vi "Export.vi"(8 "error in (no error)":errorcluster, 11 "Test Report in":refnum<class "Test Report.Event.lvclass">) -> (0 "error out":errorcluster, 3 "Test Report out":refnum<class "Test Report.Event.lvclass">)   [LabVIEW 2020, in "Caraya.lvlib" / "Test Report.Event.lvclass"]
uses:
  Test Report.Event.lvclass
  C:/projects/caraya/src/classes/Test Report/Test Report.lvclass
  Test Report.Event.lvclass/Test Report.Event.ctl
  Test Report/Test Report.lvclass
  Test Result/Test Result.lvclass
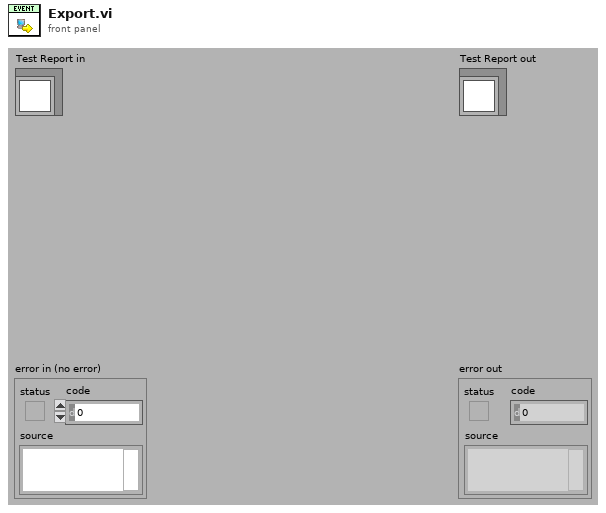
[diagram p1: front panel]
types:
  T1 = typedef "Caraya.lvlib/Test Result.lvclass/Node Results (Extended).ctl" = cluster{"Test Node":T2, "Assertions":T4[]}
  T2 = typedef "Caraya.lvlib/Test Result.lvclass/Test Node (Extended).ctl" = cluster{"Test Registration":T3, "Defined":bool, "Passed":bool, "properties":variant}
  T3 = typedef "Caraya.lvlib/Test Result.lvclass/Test Registration Data.ctl" = cluster{"Name":string, "Call Chain":string[], "Time Stamp":timestamp, "Test ID":string, "Caller ID":string}
  T4 = typedef "Caraya.lvlib/Test Result.lvclass/Assert Event Data (Extended).ctl" = cluster{"name":string, "passed":bool, "call-chain":string[], "test-error":errorcluster, "timestamp":timestamp, "assert-id":string, "test-id":string, "time":dbl, "message":string, "properties":variant, "measurements":variant, "user-defined":variant}
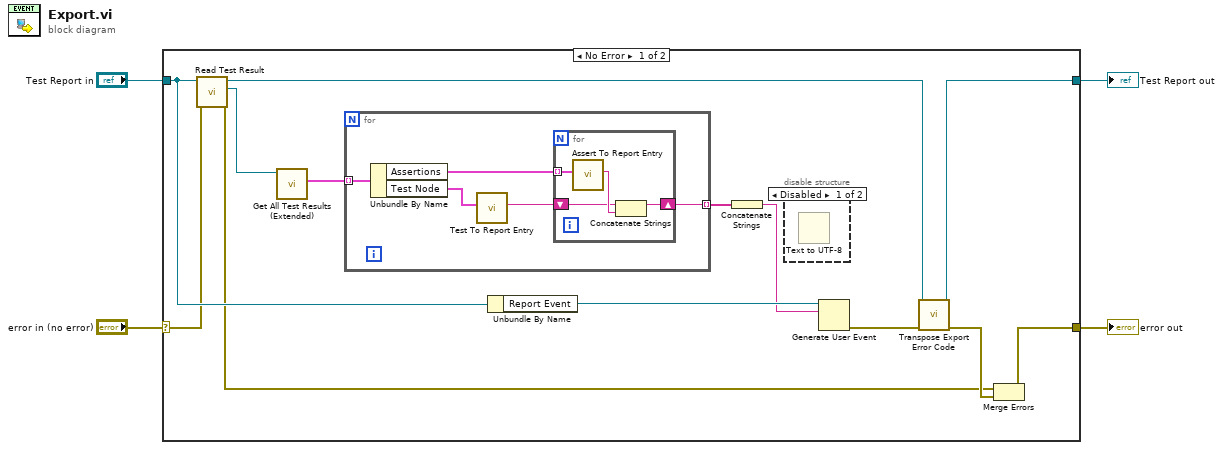
[diagram p0: block diagram]
diagram:
  n1 = case shown="No Error" "error in (no error)" {
    selector: "error in (no error)" -> [w16 w28]
    tunnel: [w13 w28] -> w3
    tunnel: [w10 w27] -> w1
    tunnel: "Test Report in" -> [w17 w27]
    frame No Error {
      n2 = call "Read Test Result.vi"("error in (no error)"=w16, "Test Report in"=w17) -> ("error out"=w12:errorcluster, "Caraya.lvlib:Test Result.lvclass"=w6:refnum<class "Test Result.lvclass">, "Test Report out"=w11:refnum<class "Test Report.Event.lvclass">)  [unwired: 7 in]
      n3 = call "Get All Test Results (Extended).vi"("Test Result in"=w6) -> ("Test Results"=w5:T1[])  [unwired: 8 in, 2 out]
      n4 = for {
        tunnel: w5 -> [w21] mode=indexing
        tunnel: [w19] -> w15 mode=indexing
        n5 = Unbundle By Name(w21) -> ("Assertions"=w18:T4[], "Test Node"=w20:T2)
        n6 = call "Test To Report Entry.vi"("Test Node"=w20) -> ("String"=w22:string)  [unwired: 9 in, 1 out]
        n7 = for {
          shift-right: [w23] -> w19
          shift-left: w22 -> [w24]
          tunnel: w18 -> [w26] mode=indexing
          n8 = call "Assert To Report Entry.vi"("Assert Event Data"=w26) -> ("String"=w25:string)  [unwired: 9 in, 1 out]
          n9 = Concatenate Strings(w24, w25) -> (w23:string)
        }
      }
      n10 = Unbundle By Name(w17) -> ("Report Event"=w9:refnum<user-event>)
      n11 = Concatenate Strings(w15) -> (w8:string)
      n12 = disable-structure shown="Disabled" {
        frame Disabled {
          n13 = Text to UTF-8() -> ()  [unwired: 3 in, 2 out]
        }
        frame Enabled {
        }
      }
      n14 = Generate User Event(user event=w9, event data cluster=w8) -> (error out=w7:errorcluster)  [unwired: 2 in, 1 out]
      n15 = call-dynamic "Transpose Export Error Code.vi"("error in (no error)"=w7, "Test Report"=w11) -> ("error out"=w14:errorcluster, "Test Report out"=w10:refnum<class "Test Report.Event.lvclass">)  [unwired: 8 in]
      n16 = Merge Errors(w12, w14) -> (w13:errorcluster)
    }
    frame Error {
    }
  }
  "error out" <- w3
  "Test Report out" <- w1
